vi "Simple Exception Handler.vi"(11 "error in (no error)":errorcluster) -> (15 "error out":errorcluster)   [LabVIEW 2015, in "LV Exceptions v1.lvlib"]
doc: "If error cluster contains an exception, it is cleared and relevant dialog box is displayed. Otherwise, value of the error cluster is forwarded to the output."
uses:
  LV Exceptions v1.lvlib
  <vilib>/Utility/error.llb/DialogTypeEnum.ctl
  <vilib>/Utility/error.llb/TagReturnType.ctl
  Exception/Exception.lvclass
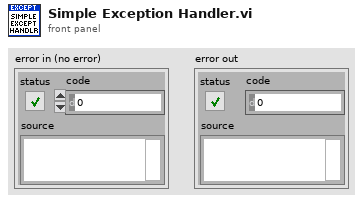
[diagram p1: front panel]
types:
  T1 = typedef "TagReturnType.ctl" = enum16{"No Tag", "<err>", "<append>"}
  T2 = typedef "DialogTypeEnum.ctl" = enum16{"no dialog", "OK message", "continue or stop message", "auto error handling dialog", "OK message + warnings", "continue/stop + warnings"}
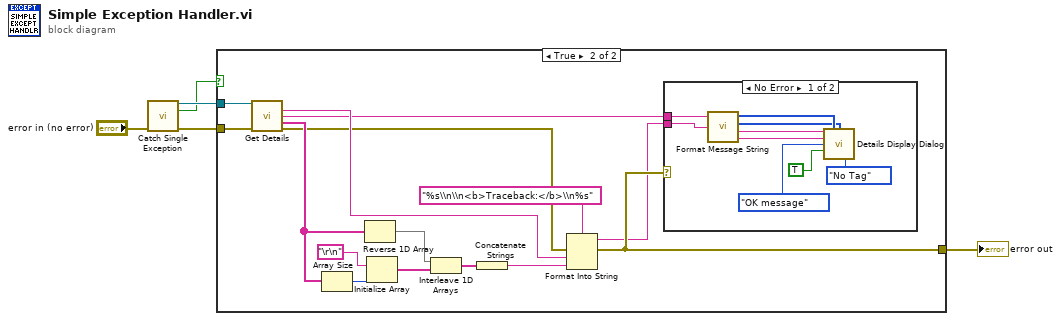
[diagram p0: block diagram]
diagram:
  n1 = call "Catch Single Exception.vi"("error in (no error)"="error in (no error)") -> ("catched exception out"=w2:refnum<class "Exception.lvclass">, "catched"=w1:bool, "error out"=w3:errorcluster)  [unwired: 12 in]
  n2 = case shown="True" w1 {
    tunnel: [w6 w21] -> w5
    tunnel: w3 -> [w6 w19]
    tunnel: w2 -> [_ w18]
    frame False {
    }
    frame True {
      n3 = call-dynamic "Get Details.vi"("exception in"=w18, "error in (no error)"=w19) -> ("message"=w9:string, "class name"=w7:string, "call chain"=w20:string[], "error out"=w8:errorcluster)  [unwired: 8 in, 2 out]
      n4 = Array Size(array=w20) -> (size(s)=w15:i32)
      n5 = Reverse 1D Array(array=w20) -> (reversed array=w12:string[])
      n6 = Initialize Array("\r\n", w15) -> (w13:string[])
      n7 = Interleave 1D Arrays(w12, w13) -> (w11:string[])
      n8 = Concatenate Strings(w11) -> (w10:string)
      n9 = Format Into String(format string="%s\\n\\n<b>Traceback:</b>\\n%s", error in=w8, w9, w10) -> (resulting string=w16:string, error out=w21:errorcluster)  [unwired: 1 in]
      n10 = case shown="No Error" w21 {
        tunnel: w16 -> [w26 _]
        tunnel: w7 -> [w27 _]
        frame No Error {
          n11 = call <vilib>:"Format Message String.vi"("Source"=w27, "Details"=w26) -> ("Bold Start"=w23:i32[], "Bold Length"=w22:i32[], "Source Out"=w25:string, "Details Out"=w24:string)  [unwired: 2 in, 1 out]
          n12 = call <vilib>:"Details Display Dialog.vi"("Source"=w25, "Start"=w23, "Length"=w22, "Details"=w24, "dialog type"=DialogTypeEnum."OK message", "Error or Warning"=TRUE, "Tag Found?"=TagReturnType."No Tag") -> ()  [unwired: 8 in, 1 out]
        }
        frame Error {
        }
      }
    }
  }
  "error out" <- w5
